vi "Compute Link Displacement Matrix.vi"(8 "error in (no error)":errorcluster, 10 "q":dbl, 11 "Link in":refnum<class "Link.lvclass">) -> (0 "error out":errorcluster, 2 "Displacement Matrix":T1, 3 "Link out":refnum<class "Link.lvclass">)   [LabVIEW 2013, in "Link.lvclass"]
uses:
  Link.lvclass
  <vilib>/Analysis/Matrix/Datatypes/RealMatrix.ctl
  Link.lvclass/Link.ctl
  <vilib>/Analysis/Matrix/Numeric/Multiply/Multiply - RM,RM.vi
  <vilib>/Analysis/Matrix/Numeric/Subtract/Subtract - RM,RM.vi
  <vilib>/Analysis/Matrix/Numeric/Add/Add - RM,RM.vi
  <vilib>/Analysis/Matrix/Numeric/Multiply/Multiply - RM,R.vi
  <vilib>/Analysis/Matrix/Numeric/Multiply/Multiply - R,RM.vi
  <vilib>/Analysis/Matrix/Numeric/Conversions/Array To Matrix - RA.vi
  <vilib>/Analysis/Matrix/Numeric/Conversions/Array To Matrix - RA2.vi
  <vilib>/Analysis/Matrix/NI_Matrix.lvlib
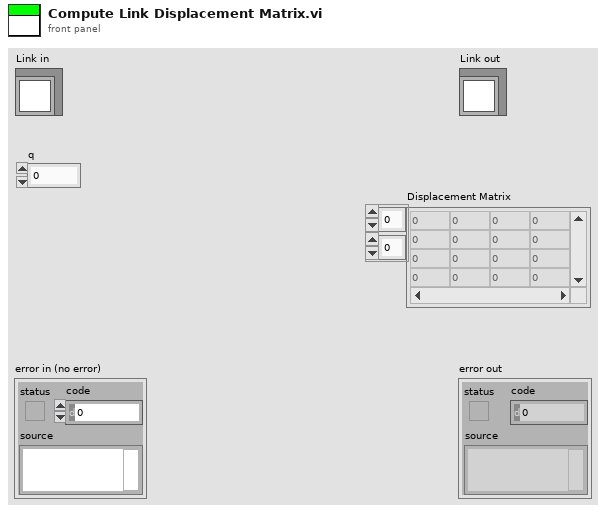
[diagram p1: front panel]
types:
  T1 = typedef "NI_Matrix.lvlib/RealMatrix.ctl" = dbl[][]
  T2 = typedef "NI_Robotics_Link.lvclass/Joint Type.ctl" = enum16{"Revolute", "Prismatic"}
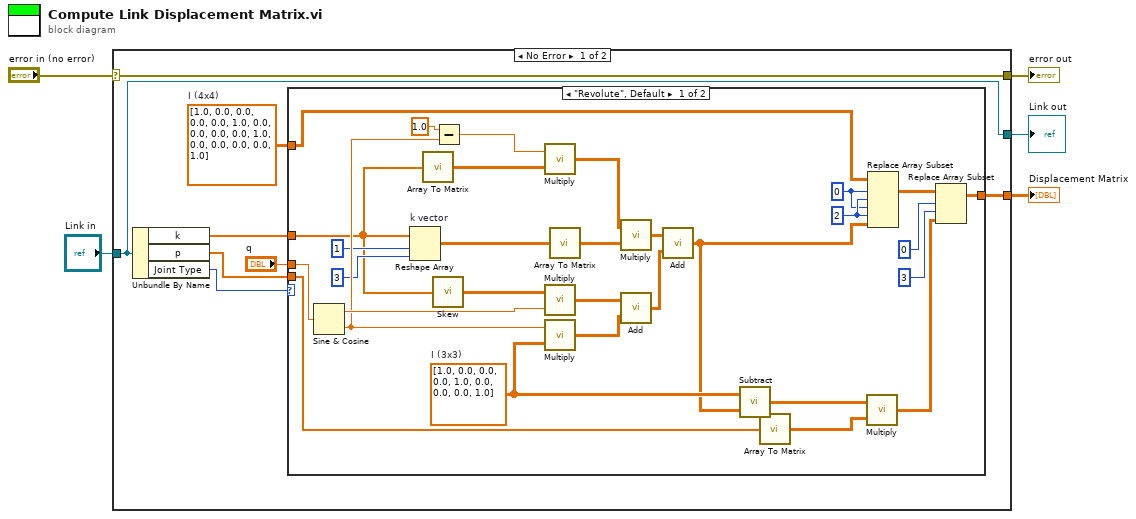
[diagram p0: block diagram]
diagram:
  n1 = case shown="No Error" "error in (no error)" {
    selector: "error in (no error)" -> [w13 w44]
    tunnel: [w13 w44] -> w4
    tunnel: [w12 w45] -> w2
    tunnel: "Link in" -> [w12 w45]
    tunnel: [w7 _] -> w1
    frame No Error {
      w8 = T1 [[1.0, 0.0, 0.0, 0.0], [0.0, 1.0, 0.0, 0.0], [0.0, 0.0, 1.0, 0.0], [0.0, 0.0, 0.0, 1.0]]  # I (4x4)
      n2 = Unbundle By Name(w12) -> ("k"=w11:dbl[], "p"=w9:dbl[], "Joint Type"=w6:T2)
      n3 = case shown="\"Revolute\", Default" w6 {
        tunnel: "q" -> [w43 _]
        tunnel: w11 -> [w14 _]
        tunnel: w9 -> [w23 _]
        tunnel: w8 -> [w17 _]
        tunnel: [w16 _] -> w7
        frame "Revolute", Default {
          w33 = 2 ("row N")
          w32 = 0 ("row 1")
          w31 = T1 [[1.0, 0.0, 0.0], [0.0, 1.0, 0.0], [0.0, 0.0, 1.0]]  # I (3x3)
          n4 = Sine & Cosine(0:w43) -> (1:w42:dbl, 2:w38:dbl)
          n5 = Reshape Array "k vector"(w14, 1 ("dimension size"), 3 ("dimension size")) -> (w24:dbl[][])
          n6 = call-poly <vilib>:"Array To Matrix.vi"("Real 1D Array"=w14) -> ("Real Matrix (Column Vector)"=w28:T1)
          n7 = call "Skew.vi"("k"=w14) -> ("M"=w15:T1)
          n8 = Subtract(x=1.0, y=w38) -> (x-y=w37:dbl)
          n9 = call-poly <vilib>:"Multiply.vi"("Real Matrix A"=w28, "Real Scalar c"=w37) -> ("c * A"=w36:T1)
          n10 = call-poly <vilib>:"Multiply.vi"("Real Scalar c"=w42, "Real Matrix A"=w15) -> ("A * c"=w40:T1)
          n11 = call-poly <vilib>:"Multiply.vi"("Real Matrix A"=w31, "Real Scalar c"=w38) -> ("c * A"=w41:T1)
          n12 = call-poly <vilib>:"Array To Matrix.vi"("Real 2D Array"=w24) -> ("Real Matrix"=w25:T1)
          n13 = call-poly <vilib>:"Multiply.vi"("Real Matrix B"=w25, "Real Matrix A"=w36) -> ("A * B"=w34:T1)
          n14 = call-poly <vilib>:"Add.vi"("Real Matrix B"=w41, "Real Matrix A"=w40) -> ("A + B"=w35:T1)
          n15 = call-poly <vilib>:"Add.vi"("Real Matrix B"=w35, "Real Matrix A"=w34) -> ("A + B"=w30:T1)
          n16 = call-poly <vilib>:"Subtract.vi"("Real Matrix B"=w30, "Real Matrix A"=w31) -> ("A - B"=w29:T1)
          n17 = call-poly <vilib>:"Array To Matrix.vi"("Real 1D Array"=w23) -> ("Real Matrix (Column Vector)"=w22:T1)
          n18 = call-poly <vilib>:"Multiply.vi"("Real Matrix B"=w22, "Real Matrix A"=w29) -> ("A * B"=w20:T1)
          n19 = Replace Array Subset(array=w17, new element=w30, index (dim 0)=w32, index (dim 1)=w33, index (dim 2)=w32, index (dim 3)=w33) -> (w21:T1)
          n20 = Replace Array Subset(array=w21, new element=w20, index (row)=0 ("disabled index (row)"), index (col)=3 ("disabled index (col)")) -> (w16:T1)
        }
        frame "Prismatic" {
          # "TODO: Implement calculation of D for prismatic joints"
        }
      }
    }
    frame Error {
    }
  }
  "error out" <- w4
  "Link out" <- w2
  "Displacement Matrix" <- w1
